vi "Jenco6173.vi"() -> (3 "PH 2":dbl=6.02)   [LabVIEW 2018]
uses:
  <vilib>/Instr/_visa.llb/VISA Configure Serial Port (Instr).vi
panel:
  out "Waveform Chart":dbl(graph)=6.02
  out "PH":dbl=6.02
  out "number 3":i32=6
  out "substring 3":string="6"
  out "number 2":i32
  out "substring 2":string="0"
  in  "offset":i32=2
  out "number":i32=2
  out "substring":string="6.02"
  out "read buffer":string="P+06.02T+023.5M+0048\r\n"
  in  "stop":bool
  in  "VISA resource name 2":refnum<visa-resource-name>="COM3"
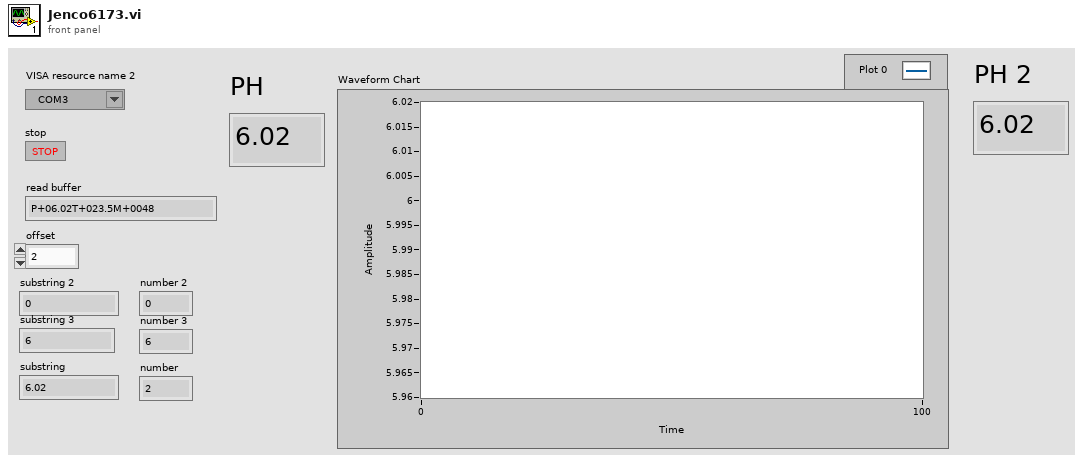
[diagram p1: front panel]
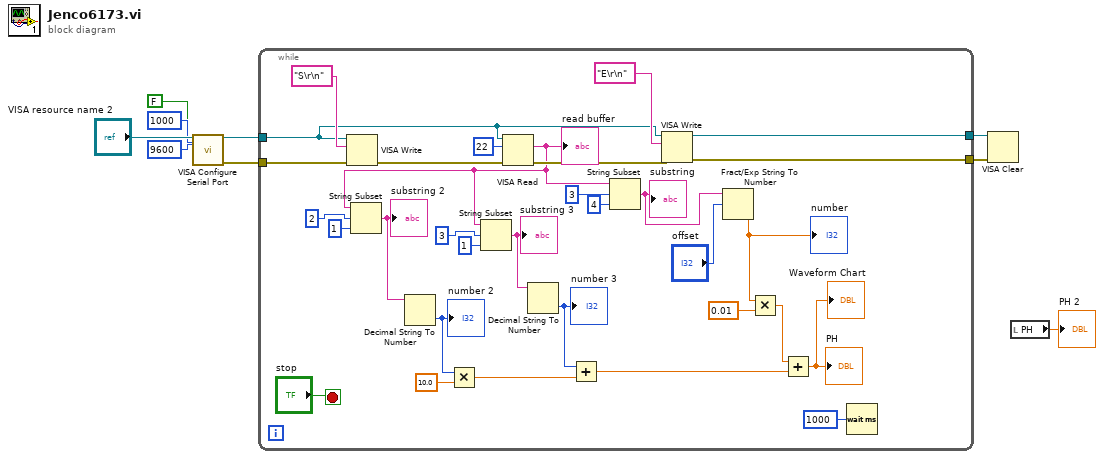
[diagram p0: block diagram]
diagram:
  n1 = call-poly "VISA Configure Serial Port"("VISA resource name"="VISA resource name 2", "timeout (10sec)"=u32 1000, "Enable Termination\nChar (T)"=FALSE ("Enable Termination\nChar (T)"), "baud rate (9600)"=u32 9600) -> ("VISA resource name out"=w9:refnum<visa-resource-name>, "error out"=w4:errorcluster)  [unwired: 10 in]
  n2 = while {
    tunnel: w9 -> [w29]
    tunnel: w4 -> [w39]
    tunnel: [w28] -> w3
    tunnel: [w27] -> w2
    stop <- "stop" stop-if-true
    n3 = VISA Write(VISA resource name=w29, write buffer="S\r\n" ("string"), error in (no error)=w39) -> (error out=w40:errorcluster)  [unwired: 2 out]
    n4 = VISA Read(VISA resource name=w29, byte count=u32 22, error in (no error)=w40) -> (read buffer=w20:string, error out=w35:errorcluster)  [unwired: 2 out]
    "read buffer" <- w20
    n5 = String Subset(string=w20, offset (0)=2, length (rest)=1 ("length (rest)")) -> (substring=w23:string)
    "substring 2" <- w23
    n6 = Decimal String To Number(string=w23) -> (number=w17:i32)  [unwired: 2 in, 1 out]
    "number 2" <- w17
    n7 = Multiply(x=w17, y=10.0) -> (x*y=w14:dbl)
    n8 = String Subset(string=w20, offset (0)=3, length (rest)=1 ("length (rest)")) -> (substring=w19:string)
    "substring 3" <- w19
    n9 = Decimal String To Number(string=w19) -> (number=w13:i32)  [unwired: 2 in, 1 out]
    "number 3" <- w13
    n10 = Add(x=w13, y=w14) -> (x+y=w12:dbl)
    n11 = String Subset(string=w20, offset (0)=3, length (rest)=4 ("length (rest)")) -> (substring=w30:string)
    "substring" <- w30
    n12 = VISA Write(VISA resource name=w29, write buffer="E\r\n" ("string"), error in (no error)=w35) -> (VISA resource name out=w28:refnum<visa-resource-name>, error out=w27:errorcluster)  [unwired: 1 out]
    n13 = Fract/Exp String To Number(string=w30, offset="offset") -> (number=w15:dbl)  [unwired: 2 in, 1 out]
    "number" <- w15
    n14 = Multiply(x=w15, y=0.01) -> (x*y=w11:dbl)
    n15 = Add(x=w11, y=w12) -> (x+y=→"PH" →"Waveform Chart":dbl)
    n16 = Wait (ms)(milliseconds to wait=u32 1000) -> ()  [unwired: 1 out]
  }
  n17 = VISA Clear(VISA resource name=w3, error in (no error)=w2) -> ()  [unwired: 2 out]
  n18 = local read "PH"() -> (→"PH 2":dbl)
